vi "Profibus_read.vi"(8 "Error in:":T1, 9 "Profibus-Addr.":i32, 10 "Var Array":T3[](array[typedef])=[{"Tag/name"="SNS_MassFlow", "Profibus Index"=4, "\nType"=enum."Float", "Profibus Slot"=0}, {"Tag/name"="SNS_Temperature", "Profibus Index"=6, "\nType"=enum."Float", "Profibus Slot"=0}], 11 "DFP2 resource name":refnum<visa-resource-name>) -> (0 "Error out:":T1 {"Status" format="%.0x"}, 1 "Error":bool, 2 "output Array":T2(array[cluster])=[{"Tag/name"="SNS_MassFlow", "\nType"=enum."Float", "Data"=0, 0, "type single"=-0.021682508}, {"Tag/name"="SNS_Temperature", "\nType"=enum."Float", "Data"=0, 0, "type single"=22.746204}], 3 "DFP2 resource name out":refnum<visa-resource-name>)   [LabVIEW 2011]
uses:
  Profibus VISA Driver/DF PROFI II.llb/CS_PB_DPV1_MSAC2_ReadReqData.ctl
  Profibus VISA Driver/DF PROFI II.llb/CS_PB_DPV1_MSAC2_AbortReqData.ctl
  Profibus VISA Driver/DF PROFI II.llb/CS_PB_DPV1_MSAC2_InitiateReqData.ctl
  Variable_cluster.ctl
panel:
  in  "Initiate data":T4={"Communication ref.:"=1, "Send timeout:"=1000, "Feat. supp. 1:"=1, "Feat. supp. 2:"=0, "Profile feat. supp. 1:"=0, "Profile feat. supp. 2:"=0, "Profile ID number:"=0, "Addional address parameter"={"S-Type"=FALSE, "S-Length:"=2, "D-Type"=FALSE, "D-Length:"=2, "Data:"=[0, 0, 0, 0]}} {"Addional address parameter"."D-Length:" format="%0.0f"; "Addional address parameter"."S-Length:" format="%0.0f"; "Addional address parameter"."Data:" format="%.0x"; "Feat. supp. 2:" format="%.0x"; "Feat. supp. 1:" format="%.0x"; "Profile feat. supp. 2:" format="%.0x"; "Profile feat. supp. 1:" format="%.0x"; "Profile ID number:" format="%.0x"; "Send timeout:" format="%0.0f"; "Communication ref.:" min=1 max=49 format="%0.0f"}
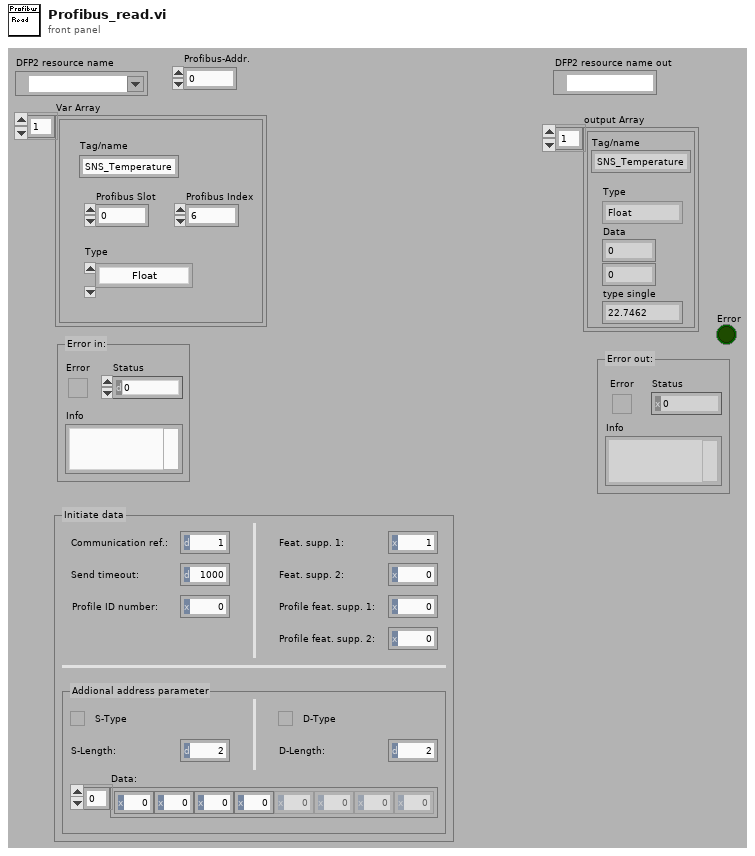
[diagram p1: front panel]
types:
  T1 = cluster{"Error":bool, "Status":i32, "Info":string}
  T2 = cluster{"Tag/name":string, "\nType":enum16{"Boolean", "Int8", "Unsigned8", "Int16", "Unsigned16", "Int32", "Unsigned32", "Float"}, "Data":u8, u16, "type single":sgl}[]
  T3 = typedef "Variable_cluster.ctl" = cluster{"Tag/name":string, "Profibus Index":i32, "\nType":enum16{"Boolean", "Int8", "Unsigned8", "Int16", "Unsigned16", "Int32", "Unsigned32", "Float"}, "Profibus Slot":i32}
  T4 = typedef "CS_PB_DPV1_MSAC2_InitiateReqData.ctl" = cluster{"Communication ref.:":u8, "Send timeout:":u16, "Feat. supp. 1:":u8, "Feat. supp. 2:":u8, "Profile feat. supp. 1:":u8, "Profile feat. supp. 2:":u8, "Profile ID number:":u16, "Addional address parameter":cluster{"S-Type":bool, "S-Length:":u8, "D-Type":bool, "D-Length:":u8, "Data:":u8[]}}
  T5 = typedef "CS_PB_DPV1_MSAC2_AbortReqData.ctl" = cluster{"Communication ref.:":u8, "Subnet:":u8, "Instance &\nReasoncode:":u8, "Additional detail:":u16}
  T6 = typedef "CS_PB_DPV1_MSAC2_InitiateConData.ctl" = cluster{"Communication ref.:":u8, "Remote add.:":u8, "Feat. supp. 1:":u8, "Feat. supp. 2:":u8, "Profile feat. supp. 1:":u8, "Profile feat. supp. 2:":u8, "Profile ID number:":u16, "Addional address parameter":cluster{"S-Type":bool, "S-Length:":u8, "D-Type":bool, "D-Length:":u8, "Data:":u8[]}, "Max length data unit:":u8}
  T7 = typedef "CS_PB_DPV1_MSAC2_ErrorData.ctl" = cluster{"Communication ref.:":u8, "Remote address:":u8, "Error decode:":u8, "Error code 1:":u8, "Error code 2:":u8}
  T8 = typedef "CS_PB_DPV1_MSAC2_AbortIndData.ctl" = cluster{"Remote address:":u8, "Response SAP:":u8, "Locally generated":bool, "Subnet:":u8, "Instance:":u8, "Reasoncode:":u8, "Additional detail:":u16}
  T9 = cluster{"Initiate data":T6, "Error data":T7, "Abort data":T8}
  T10 = typedef "CS_PB_DPV1_MSAC2_ReadReqData.ctl" = cluster{"Communication ref.:":u8, "Slot number:":u8, "Index:":u8, "Length:":u8}
  T11 = enum16{"Boolean", "Int8", "Unsigned8", "Int16", "Unsigned16", "Int32", "Unsigned32", "Float"}
  T12 = typedef "CS_PB_DPV1_MSAC2_ReadConData.ctl" = cluster{"Communication ref.:":u8, "Length:":u8, "Data:":u8[]}
  T13 = typedef "CS_PB_DPV1_AbortIndData.ctl" = cluster{"Remote address:":u8, "Response SAP:":u8, "Locally generated":bool, "Subnet:":u8, "Instance:":u8, "Reasoncode:":u8, "Additional detail:":u16}
  T14 = typedef "CS_PB_DPV1_ErrorData.ctl" = cluster{"Communication ref.:":u8, "Remote address:":u8, "Error decode:":u8, "Error code 1:":u8, "Error code 2:":u8}
  T15 = cluster{"Read data":T12, "Abort data":T13, "Error data":T14}
  T16 = cluster{"Tag/name":string, "\nType":enum16{"Boolean", "Int8", "Unsigned8", "Int16", "Unsigned16", "Int32", "Unsigned32", "Float"}, "Data":u8, u16, "type single":sgl}
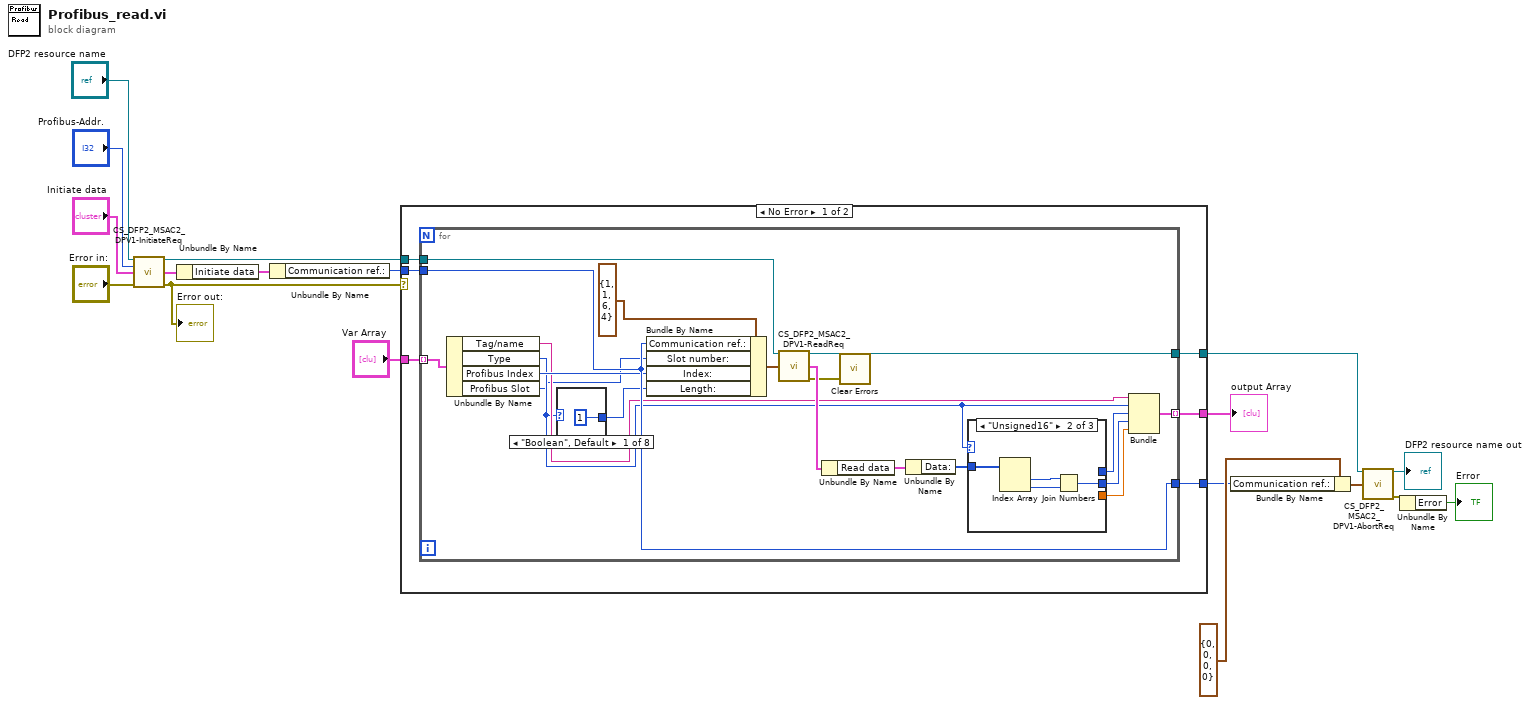
[diagram p0: block diagram]
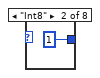
[diagram p2: hidden frame]
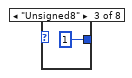
[diagram p3: hidden frame]
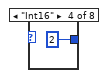
[diagram p4: hidden frame]
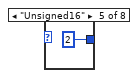
[diagram p5: hidden frame]
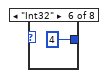
[diagram p6: hidden frame]
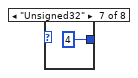
[diagram p7: hidden frame]
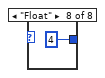
[diagram p8: hidden frame]
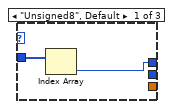
[diagram p9: hidden frame]
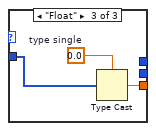
[diagram p10: hidden frame]
diagram:
  n1 = call "CS_DFP2_MSAC2_DPV1-InitiateReq.vi"("DFP2 resource name"="DFP2 resource name", "Profibus-Addr."="Profibus-Addr.", "Initiate data"="Initiate data", "Error in:"="Error in:") -> ("DFP2 resource name out"=w17:refnum<visa-resource-name>, "DPV1-Initiate"=w15:T9, "Error out:"=w16:T1)  [unwired: 8 in, 1 out]
  "Error out:" <- w16
  n2 = Unbundle By Name(w15) -> ("Initiate data"=w14:T6)
  n3 = Unbundle By Name(w14) -> ("Communication ref.:"=w13:u8)
  n4 = case shown="No Error" w16 {
    tunnel: w17 -> [w24 w62]
    tunnel: w13 -> [w23 w61]
    tunnel: [w22 w62] -> w7
    tunnel: [w21 w61] -> w4
    tunnel: "Var Array" -> [w20 _]
    tunnel: [w19 _] -> w11
    frame No Error {
      n5 = for {
        tunnel: w24 -> [w43]
        tunnel: w23 -> [w37]
        tunnel: [w38] -> w22
        tunnel: [w37] -> w21
        tunnel: w20 -> [w36] mode=indexing
        tunnel: [w27] -> w19 mode=indexing
        n6 = Unbundle By Name(w36) -> ("Tag/name"=w32:string, "Type"=w31:T11, "Profibus Index"=w34:i32, "Profibus Slot"=w25:i32)
        n7 = case shown="\"Boolean\", Default" w31 {
          tunnel: [u8 1 ("Length:") u8 1 ("Length:") u8 1 ("Length:") u8 2 ("Length:") u8 2 ("Length:") u8 4 ("Length:") u8 4 ("Length:") u8 4 ("Length:")] -> w33
          frame "Boolean", Default {
          }
          frame "Int8" {
          }
          frame "Unsigned8" {
          }
          frame "Int16" {
          }
          frame "Unsigned16" {
          }
          frame "Int32" {
          }
          frame "Unsigned32" {
          }
          frame "Float" {
          }
        }
        n8 = Bundle By Name(cluster=T10 {"Communication ref.:"=1, "Slot number:"=1, "Index:"=6, "Length:"=4} ("Read data"), "Communication ref.:"=w37, "Slot number:"=w25, "Index:"=w34, "Length:"=w33) -> (w39:T10)
        n9 = call "CS_DFP2_MSAC2_DPV1-ReadReq.vi"("DFP2 resource name"=w43, "Read data"=w39) -> ("DFP2 resource name out"=w38:refnum<visa-resource-name>, "DPV1-Read"=w42:T15, "Error out:"=w26:T1)  [unwired: 10 in, 1 out]
        n10 = Unbundle By Name(w42) -> ("Read data"=w41:T12)
        n11 = call <vilib>:"Clear Errors.vi"("error in (no error)"=w26) -> ()  [unwired: 6 in, 1 out]
        n12 = Unbundle By Name(w41) -> ("Data:"=w35:u8[])
        n13 = case shown="\"Unsigned16\"" w31 {
          tunnel: w35 -> [w53 w57 w59]
          tunnel: [w52 _ _] -> w30
          tunnel: [_ w54 _] -> w29
          tunnel: [_ _ w58] -> w28
          frame "Unsigned8", Default {
            n14 = Index Array(array=w53) -> (element=w52:u8)  [unwired: 1 in]
          }
          frame "Unsigned16" {
            n15 = Index Array(array=w57) -> (element #1=w56:u8, element #2=w55:u8)  [unwired: 2 in]
            n16 = Join Numbers(hi=w56, lo=w55) -> ((hi.lo)=w54:u16)
          }
          frame "Float" {
            w60 = sgl 0.0  # type single
            n17 = Type Cast(type=w60, x=w59) -> (*(type *) &x=w58:sgl)
          }
        }
        n18 = Bundle("Tag/name"=w32, "Type"=w31, "Data"=w30, w29, "type single"=w28) -> (w27:T16)  [unwired: 1 in]
      }
    }
    frame Error {
    }
  }
  "output Array" <- w11
  n19 = Bundle By Name(cluster=T5 {"Communication ref.:"=0, "Subnet:"=0, "Instance &\nReasoncode:"=0, "Additional detail:"=0} ("Abort data"), "Communication ref.:"=w4) -> (w3:T5)
  n20 = call "CS_DFP2_MSAC2_DPV1-AbortReq.vi"("DFP2 resource name"=w7, "Abort data"=w3) -> ("DFP2 resource name out"=→"DFP2 resource name out":refnum<visa-resource-name>, "Error out:"=w2:T1)  [unwired: 10 in, 2 out]
  n21 = Unbundle By Name(w2) -> ("Error"=→"Error":bool)
